vi "Configure GPIO Timestamp DMA FIFO.vi"(0 "fpga interface in":refnum<k20>, 7 "gpio timestamp dma fifo depth (elements)":u32=10240, 11 "error in (no error)":errorcluster) -> (4 "fpga interface out":refnum<k20>, 15 "error out":errorcluster)   [LabVIEW 2023, in "GettingStarted_Common_148X_Host.lvlib"]
uses:
  GettingStarted_Common_148X_Host.lvlib
  Types/148x_Common_FPGA_Reference.ctl
  <vilib>/rvi/interface/common/niFpgaWaitOnOcc.vi
  <vilib>/Utility/error.llb/Error Cluster From Error Code.vi
  <vilib>/rvi/interface/nirviMethod/nirviMethod.xnode
  <vilib>/FPGAPlugInAG/Dynamic/niLvFpga_ConfigureFifo_Dynamic.vi
  <vilib>/rvi/errors/niLvFpgaMergeErrorWithErrorCode.vi
  <vilib>/FPGAPlugInAG/Dynamic/niLvFpga_StartFifo_Dynamic.vi
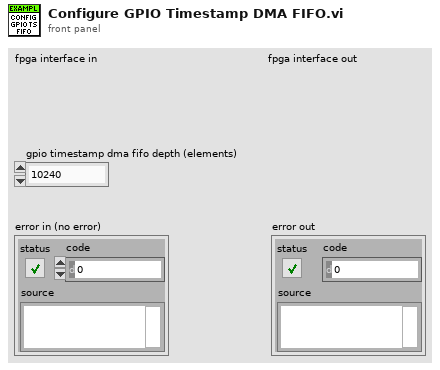
[diagram p1: front panel]
types:
  T1 = typedef "GettingStarted_Common_148X_Host.lvlib/148x_Common_FPGA_Reference.ctl" = refnum<k20>
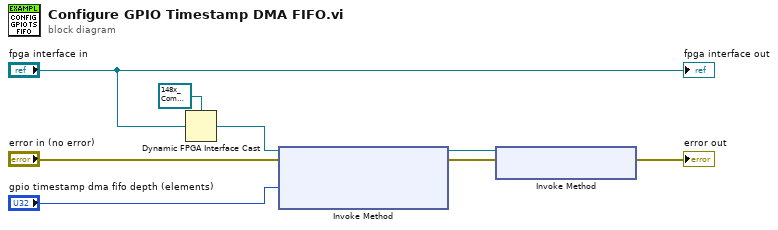
[diagram p0: block diagram]
diagram:
  n1 = Dynamic FPGA Interface Cast(Session In=T1 refnum ("FPGA VI Reference Out"), Type="fpga interface in") -> (Session Out=w6:T1)
  n2 = xnode "Invoke Method"("FPGA VI Reference In"=w6, "error in"="error in (no error)", "Requested Depth"="gpio timestamp dma fifo depth (elements)") -> ("FPGA VI Reference Out"=w5:T1, "error out"=w3:errorcluster)  [unwired: 1 out]
  n3 = xnode "Invoke Method"("FPGA VI Reference In"=w5, "error in"=w3) -> ("error out"=→"error out":errorcluster)  [unwired: 1 out]
  "fpga interface out" <- "fpga interface in"
